vi "m1m3_monitorCommand_Start.vi"(8 "error in (no error)":errorcluster, 11 "command_Start_Ctl":T1={"Start"=FALSE, "SettingsToApply"="                                                                                                                                                                                                                                                                "}) -> (0 "error out":errorcluster, 2 "function return":i32, 3 "command_Start_Ctl out":T1={"Start"=FALSE, "SettingsToApply"="                                                                                                                                                                                                                                                                "})   [LabVIEW 2016, in "SALLV_m1m3.lvlib"]
doc: "int m1m3_shm_monitorCommand_StartLV(m1m3_command_StartLV *command_Start_Ctl );"
uses:
  SALLV_m1m3.lvlib
  DataTypes/command_Start.ctl
  SALLV_m1m3.so
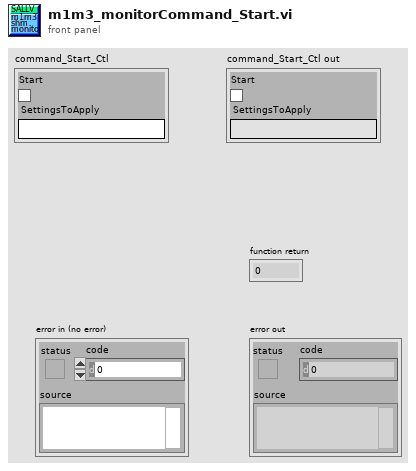
[diagram p1: front panel]
types:
  T1 = typedef "SALLV_m1m3.lvlib/command_Start.ctl" = cluster{"Start":bool, "SettingsToApply":string}
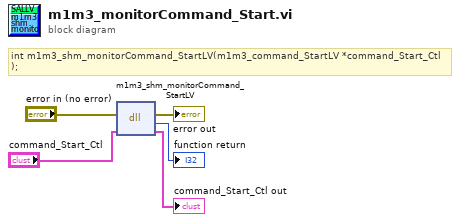
[diagram p0: block diagram]
diagram:
  # "int m1m3_shm_monitorCommand_StartLV(m1m3_command_StartLV *command_Start_Ctl );"
  n1 = dll-call lib="opt/CODE/SALLV_m1m3/SALLV_m1m3.*" fn="m1m3_shm_monitorCommand_StartLV"(error in="error in (no error)", "command_Start_Ctl"="command_Start_Ctl") -> (error out=→"error out":errorcluster, →"function return":i32, "command_Start_Ctl"=→"command_Start_Ctl out":T1)  [unwired: 2 in, 1 out]
